vi "input_channel_producer.vi"(7 "Index":i32, 8 "error in (no error)":errorcluster, 9 "aData Out":dbl[][](array[numeric]), 10 "Q":refnum<queue>) -> (0 "error out":errorcluster)   [LabVIEW 2025, in "LabJackEKG.lvlib"]
uses:
  LabJackEKG.lvlib
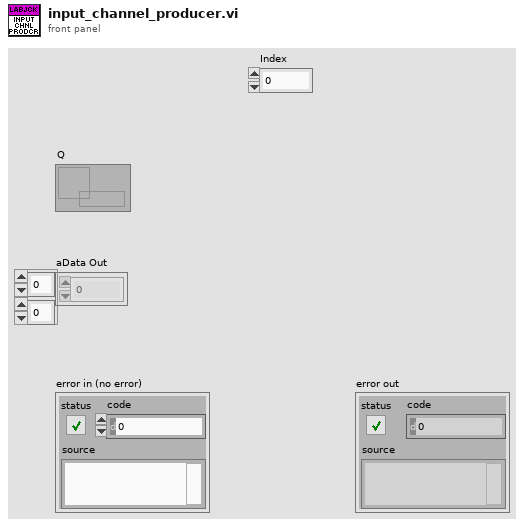
[diagram p1: front panel]
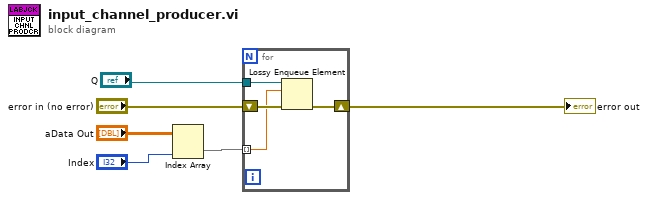
[diagram p0: block diagram]
diagram:
  n1 = Index Array(array="aData Out", index (col)="Index") -> (element=w3:dbl[])  [unwired: 1 in]
  n2 = for {
    tunnel: "Q" -> [w10]
    shift-right: [w9] -> w6
    shift-left: "error in (no error)" -> [w8]
    tunnel: w3 -> [w7] mode=indexing
    n3 = Lossy Enqueue Element(queue=w10, element=w7, error in (no error)=w8) -> (error out=w9:errorcluster)  [unwired: 3 out]
  }
  "error out" <- w6
